vi "CRYAna Auto Delay.vi"(4 "Additive Info":T3, 6 "Distance Unit":u16, 7 "Polarity":bool, 8 "Fs":dbl, 9 "Response":dbl[](array[numeric]), 10 "Stimulus":dbl[](array[numeric]), 11 "Channel Name":string) -> (1 "Result Response":dbl[](array[numeric]), 2 "Value Out":T1[](array[typedef]) {"Z data" items=["dB", "Lin"]; "X data" items=["dB", "Lin"]; "Y data" items=["dB", "Lin"]; "Z dB ref" format="%.1f"; "Z axis" items=["Log", "Lin"]; "X dB ref" format="%.1f"; "X axis" items=["Log", "Lin"]; "Y axis" items=["Log", "Lin"]; "Y dB ref" format="%.1f"; "Curve"."z" format="%.2f"; "Curve"."y" format="%.2f"; "Curve"."x" format="%.2f"}, 3 "delay [s]":dbl format="%.2f")   [LabVIEW 2013]
uses:
  Typedef Control/CRYData Cluster.ctl
panel:
  out "array of clusters":T2(array[cluster])
  in  "Datum":T1={"Name"="", "Curve"=[], "X data"=1, "Y data"=1, "Z data"=1, "X axis"=0, "Y axis"=1, "Z axis"=1, "X unit"="", "Y unit"="", "Z unit"="", "X dB ref"=1.0, "Y dB ref"=1.0, "Z dB ref"=1.0, "single val"=FALSE, "protected"=FALSE, "display X"=TRUE, "display Y"=FALSE, "display Z"=TRUE, "Test Info"="", "Step No."=0, "Plot Settings"={"Color"=0, "Interpolation"=0, "Point Style"=0, "Line Style"=0, "Point Color"=0, "Line Width"=0, "Bar Plot Style"=0, "Fill To"=0}, "AutoProtect"=FALSE} {"Z data" items=["dB", "Lin"]; "X data" items=["dB", "Lin"]; "Y data" items=["dB", "Lin"]; "Z dB ref" format="%.1f"; "Z axis" items=["Log", "Lin"]; "X dB ref" format="%.1f"; "X axis" items=["Log", "Lin"]; "Y axis" items=["Log", "Lin"]; "Y dB ref" format="%.1f"; "Curve"."z" format="%.2f"; "Curve"."y" format="%.2f"; "Curve"."x" format="%.2f"}
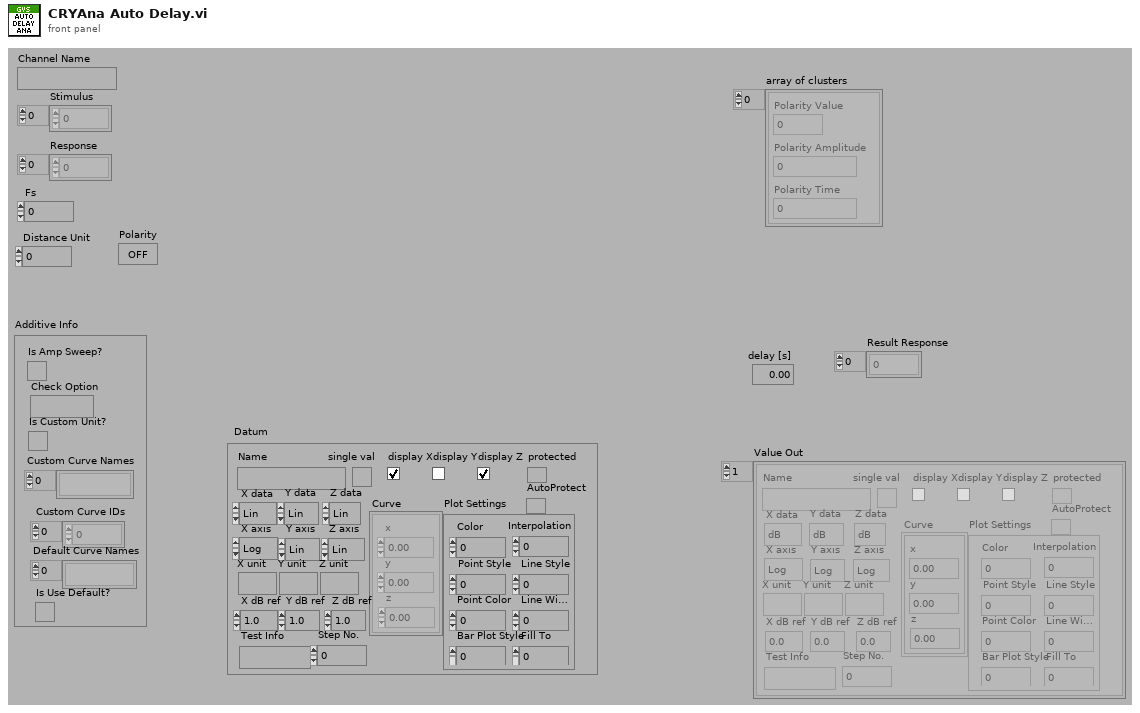
[diagram p1: front panel]
types:
  T1 = typedef "CRYData Cluster.ctl" = cluster{"Name":string, "Curve":cluster{"x":dbl, "y":dbl, "z":dbl}[], "X data":u16, "Y data":u16, "Z data":u16, "X axis":u16, "Y axis":u16, "Z axis":u16, "X unit":string, "Y unit":string, "Z unit":string, "X dB ref":dbl, "Y dB ref":dbl, "Z dB ref":dbl, "single val":bool, "protected":bool, "display X":bool, "display Y":bool, "display Z":bool, "Test Info":string, "Step No.":i32, "Plot Settings":cluster{"Color":u32, "Interpolation":u8, "Point Style":u8, "Line Style":u8, "Point Color":u32, "Line Width":u8, "Bar Plot Style":u8, "Fill To":i16}, "AutoProtect":bool}
  T2 = cluster{"Polarity Value":dbl, "Polarity Amplitude":dbl, "Polarity Time":dbl}[]
  T3 = cluster{"Is Amp Sweep?":bool, "Check Option":string, "Is Custom Unit?":bool, "Custom Curve Names":string[], "Custom Curve IDs":i32[], "Default Curve Names":string[], "Is Use Default?":bool}
  T4 = cluster{"display X":bool, "display Y":bool, "display Z":bool}[]
  T5 = cluster{"X unit":string, "X data":u16, "Y unit":string, "X data":u16, "Y unit":string, "X data":u16, "dB ref In":dbl}[]
  T6 = typedef "CRYAnalysis CurveName Cluster.ctl" = cluster{"Custom Curve Name":string, "Custom Curve ID":i32, "Default Curve Name":string}[]
  T7 = cluster{"Custom Curve Name":string, "Custom Curve ID":i32, "Default Curve Name":string}
  T8 = cluster{"X unit":string, "X data":u16, "Y unit":string, "X data":u16, "Y unit":string, "X data":u16, "dB ref In":dbl}
  T9 = cluster{"display X":bool, "display Y":bool, "display Z":bool}
  T10 = cluster{"Polarity Amplitude":dbl, "Polarity Value":dbl, "Polarity Time":dbl}[]
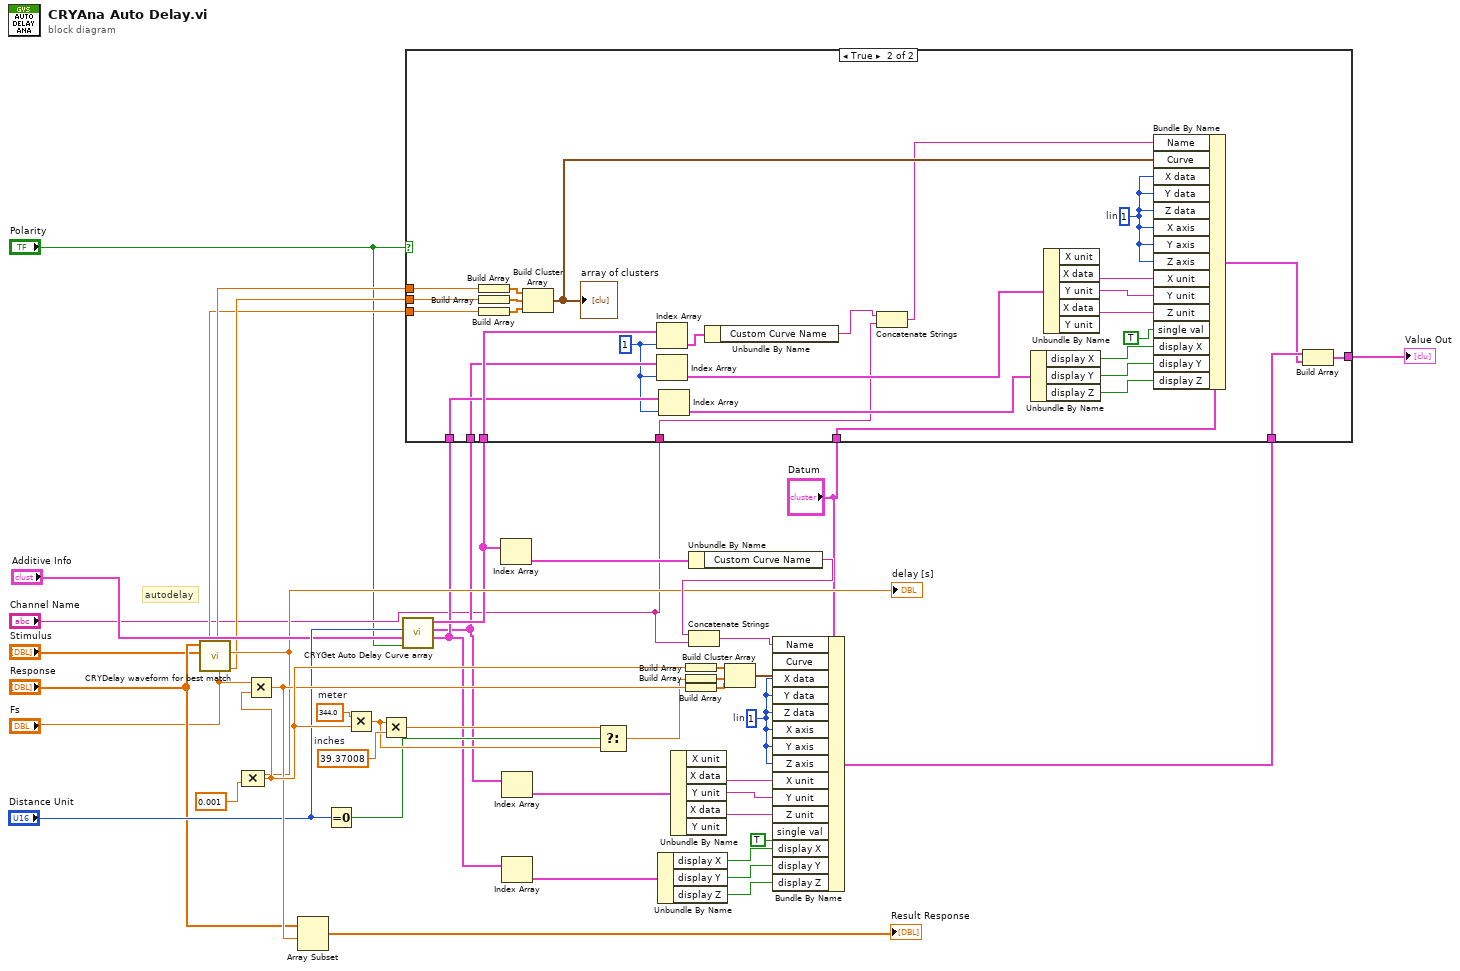
[diagram p0: block diagram]
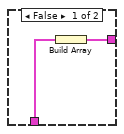
[diagram p2: hidden frame]
diagram:
  w35 = 39.37008  # inches
  w36 = 344.0  # meter
  w41 = u16 1  # lin
  # "autodelay"
  n1 = call "CRYDelay waveform for best match.vi"("Sampling rate (Hz)"="Fs", "stimulus waveform"="Stimulus", "Recorded waveform"="Response") -> ("Polarity Value"=w13:dbl, "Delay (ms)"=w16:dbl, "Polarity Amplitude"=w12:dbl, "Polarity Time"=w11:dbl)  [unwired: 5 out]
  "delay [s]" <- w16
  n2 = Compound Arithmetic op=MULTIPLY(w16, 0.001) -> (w43:dbl)
  n3 = Multiply(x="Fs", y=w43) -> (x*y=w42:dbl)
  n4 = Array Subset(array="Response", index=w42) -> (→"Result Response":dbl[])  [unwired: 1 in]
  n5 = Equal To 0?(x="Distance Unit") -> (x = 0?=w23:bool)
  n6 = Multiply(x=w36, y=w43) -> (x*y=w33:dbl)
  n7 = Multiply(x=w33, y=w35) -> (x*y=w34:dbl)
  n8 = call "CRYGet Auto Delay Curve array.vi"("Polarity"="Polarity", "Additive Info"="Additive Info", "Distance Unit"="Distance Unit") -> ("Value Display Array"=w6:T4, "Value Unit Info Out"=w5:T5, "Curve Info Array Out"=w7:T6)  [unwired: 6 in]
  n9 = Index Array(array=w7) -> (element=w21:T7)  [unwired: 1 in]
  n10 = Index Array(array=w5) -> (element=w10:T8)  [unwired: 1 in]
  n11 = Index Array(array=w6) -> (element=w9:T9)  [unwired: 1 in]
  n12 = Select(t=w34, s=w23, f=w33) -> (s? t:f=w32:dbl)
  n13 = Unbundle By Name(w9) -> ("display X"=w27:bool, "display Y"=w26:bool, "display Z"=w25:bool)
  n14 = Unbundle By Name(w10) -> ("X unit"=w30:string, "Y unit"=w29:string, "Y unit"=w28:string)  [unwired: 2 out]
  n15 = Build Array(w43) -> (w38:dbl[])
  n16 = Build Array(w32) -> (w39:dbl[])
  n17 = Build Array(w42) -> (w40:dbl[])
  n18 = Unbundle By Name(w21) -> ("Custom Curve Name"=w20:string)
  n19 = Concatenate Strings(w20, "Channel Name") -> (w22:string)
  n20 = Build Cluster Array(w38, w39, w40) -> (w37:cluster{dbl, dbl, dbl}[])
  n21 = Bundle By Name(cluster="Datum", "Name"=w22, "Curve"=w37, "X data"=w41, "Y data"=w41, "Z data"=w41, "X axis"=w41, "Y axis"=w41, "Z axis"=w41, "X unit"=w30, "Y unit"=w29, "Z unit"=w28, "single val"=TRUE ("Bundle Element"), "display X"=w27, "display Y"=w26, "display Z"=w25) -> (w3:T1)
  n22 = case shown="True" "Polarity" {
    tunnel: w13 -> [_ w47]
    tunnel: w12 -> [_ w48]
    tunnel: w11 -> [_ w72]
    tunnel: "Datum" -> [_ w52]
    tunnel: w7 -> [_ w63]
    tunnel: w6 -> [_ w62]
    tunnel: w5 -> [_ w61]
    tunnel: "Channel Name" -> [_ w54]
    tunnel: w3 -> [w46 w51]
    tunnel: [w45 w49] -> w2
    frame False {
      n23 = Build Array(w46) -> (w45:T1[])
    }
    frame True {
      w57 = 1 ("index")
      w71 = u16 1  # lin
      n24 = Build Array(w48) -> (w75:dbl[])
      n25 = Build Array(w47) -> (w74:dbl[])
      n26 = Build Array(w72) -> (w73:dbl[])
      n27 = Build Cluster Array(w75, w74, w73) -> (w58:T10)
      "array of clusters" <- w58
      n28 = Index Array(array=w63, index=w57) -> (element=w56:T7)
      n29 = Index Array(array=w61, index=w57) -> (element=w60:T8)
      n30 = Index Array(array=w62, index=w57) -> (element=w59:T9)
      n31 = Unbundle By Name(w56) -> ("Custom Curve Name"=w55:string)
      n32 = Concatenate Strings(w55, w54) -> (w53:string)
      n33 = Unbundle By Name(w59) -> ("display X"=w66:bool, "display Y"=w65:bool, "display Z"=w64:bool)
      n34 = Unbundle By Name(w60) -> ("X unit"=w69:string, "Y unit"=w68:string, "Y unit"=w67:string)  [unwired: 2 out]
      n35 = Bundle By Name(cluster=w52, "Name"=w53, "Curve"=w58, "X data"=w71, "Y data"=w71, "Z data"=w71, "X axis"=w71, "Y axis"=w71, "Z axis"=w71, "X unit"=w69, "Y unit"=w68, "Z unit"=w67, "single val"=TRUE ("Bundle Element"), "display X"=w66, "display Y"=w65, "display Z"=w64) -> (w50:T1)
      n36 = Build Array(w51, w50) -> (w49:T1[])
    }
  }
  "Value Out" <- w2
